vi "ProcessVi.vi"(1 "Refnum in":refnum<k20>, 2 "Array In":u8[](array[numeric]), 3 "ModbusSend":T1, 4 "Data":u16[](array[numeric])) -> (0 "Array out":u8[](array[numeric]))   [LabVIEW 2018]
uses:
  Commands/Address.ctl
  <vilib>/Utility/error.llb/Error Cluster From Error Code.vi
  <vilib>/rvi/errors/niLvFpgaAdjustHostInterfaceError.vi
  <vilib>/rvi/interface/nirviMethod/nirviMethod.xnode
  <vilib>/FPGAPlugInAG/Dynamic/niLvFpga_WriteFifo_Dynamic.vi
  <vilib>/rvi/errors/niLvFpgaMergeErrorWithErrorCode.vi
  Common_FPGA_Modbus/FPGAModbus.lvlib
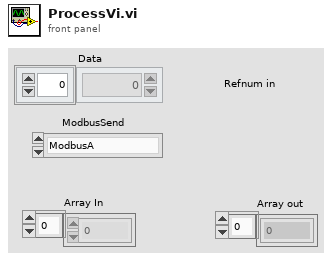
[diagram p1: front panel]
types:
  T1 = typedef "Address.ctl" = enum16{"ModbusA", "ModbusB", "ModbusC", "ModbusD", "ModbusE"}
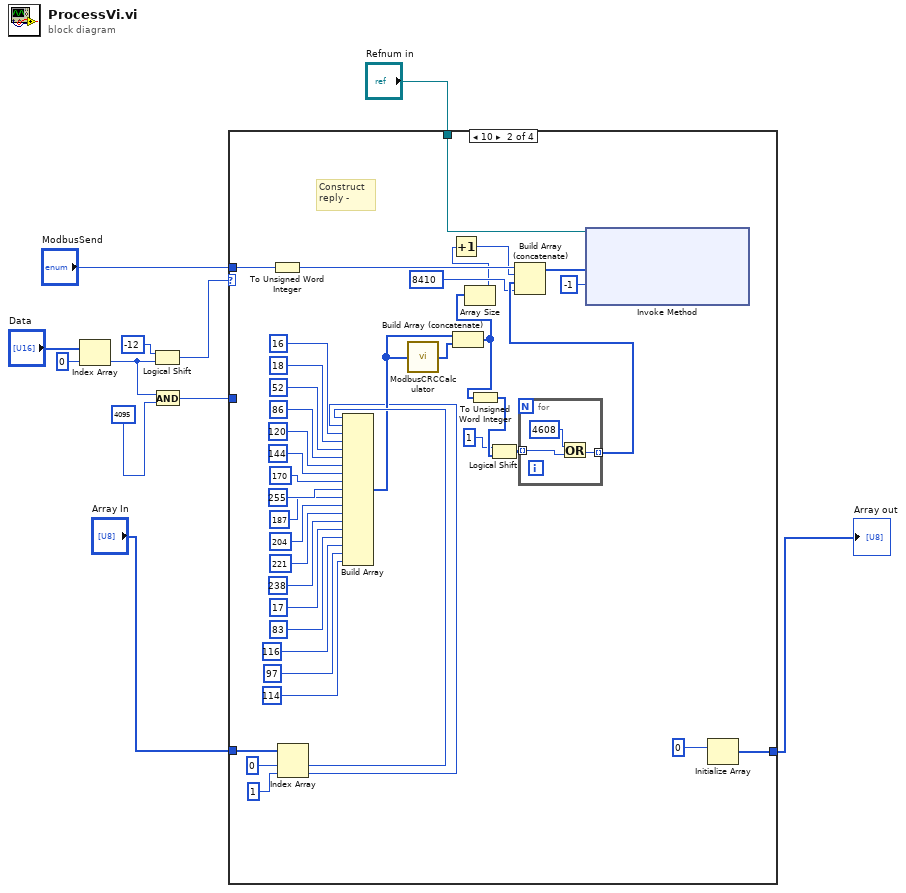
[diagram p0: block diagram]
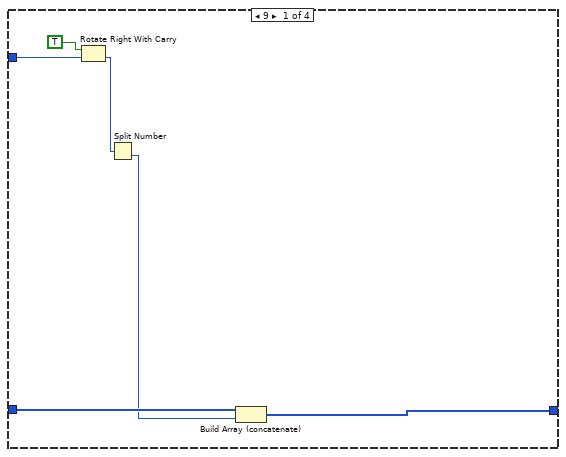
[diagram p2: hidden frame]
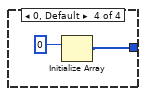
[diagram p4: hidden frame]
diagram:
  n1 = Index Array(array="Data", index=u16 0 ("element")) -> (element=w5:u16)
  n2 = Logical Shift(y=i8 -12 ("x << y"), x=w5) -> (x << y=w8:u16)
  n3 = And(x=w5, y=u16 4095 ("x .and. y?")) -> (x .and. y?=w3:u16)
  n4 = case shown="10" w8 {
    tunnel: "Refnum in" -> [_ w56 _ _]
    tunnel: "ModbusSend" -> [_ w54 _ _]
    tunnel: w3 -> [w15 _ _ _]
    tunnel: "Array In" -> [w17 w51 w60 _]
    tunnel: [w16 w52 w60 w62] -> w1
    frame 9 {
      n5 = Rotate Right With Carry(2:w15, 3:TRUE) -> (0:w14:u16)  [unwired: 1 out]
      n6 = Split Number(x=w14) -> (lo(x)=w13:u8)  [unwired: 1 out]
      n7 = Build Array (concatenate)(w17, w13) -> (w16:u8[])
    }
    frame 10 {
      # "Construct \nreply -"
      n8 = To Unsigned Word Integer(number=w54) -> (unsigned 16bit integer=w49:u16)
      n9 = Index Array(array=w51, index #1=u8 0 ("element"), index #2=1 ("index")) -> (element #1=w46:u8, element #2=w18:u8)
      n10 = Build Array(w46, w18, u8 16 ("element"), u8 18 ("element"), u8 52 ("element"), u8 86 ("element"), u8 120 ("element"), u8 144 ("element"), u8 170 ("element"), u8 255 ("element"), u8 187 ("element"), u8 204 ("element"), u8 221 ("element"), u8 238 ("element"), u8 17 ("element"), u8 83 ("element"), u8 116 ("element"), u8 97 ("element"), u8 114 ("element")) -> (w27:u8[])
      n11 = call "ModbusCRCCalculator.vi"("Input"=w27) -> ("Output"=w28:u8[])
      n12 = Build Array (concatenate)(w27, w28) -> (w26:u8[])
      n13 = Array Size(array=w26) -> (size(s)=w20:i32)
      n14 = Increment(x=w20) -> (x+1=w19:i32)
      n15 = To Unsigned Word Integer(number=w26) -> (unsigned 16bit integer=w25:u16[])
      n16 = Logical Shift(y=i16 1, x=w25) -> (x << y=w22:u16[])
      n17 = for {
        tunnel: [w58] -> w23 mode=indexing
        tunnel: w22 -> [w59] mode=indexing
        n18 = Or(x=u16 4608 ("x .or. y?"), y=w59) -> (x .or. y?=w58:u16)
      }
      n19 = Build Array (concatenate)(w49, w19, w23, 8410) -> (w48:i32[])
      n20 = xnode "Invoke Method"("FPGA VI Reference In"=w56, "Data"=w48, "Timeout (ms)"=-1) -> ()  [unwired: 1 in, 3 out]
      n21 = Initialize Array(u8 0 ("element")) -> (w52:u8[])  [unwired: 1 in]
    }
    frame 11 {
    }
    frame 0, Default {
      n22 = Initialize Array(u8 0 ("element")) -> (w62:u8[])  [unwired: 1 in]
    }
  }
  "Array out" <- w1
